vi "GPS.vi"() -> ()   [LabVIEW 2020]
uses:
  <vilib>/Instr/_visa.llb/VISA Configure Serial Port (Instr).vi
panel:
  out "before substring 10":string
  out "before substring 9":string
  out "before substring 8":string
  out "before substring 7":string
  out "before substring 6":string
  out "before substring 5":string
  out "before substring 4":string
  out "before substring 3":string
  out "before substring 2":string
  out "before substring":string
  in  "VISA resource name":refnum<visa-resource-name>
  in  "label":string
  in  "marker color":string
  in  "WebBrowser":refnum<k7>(container)
  in  "Map Format":string(combo)="roadmap"
  in  "Size X":dbl=450.0
  in  "Size Y":dbl=650.0
  in  "Zoom":sgl=16.0 format="%#.1g"
  in  "Longitude":dbl=-1.3070000000000026 format="%#.6g"
  in  "Latitude":dbl=51.4062 format="%#.6g"
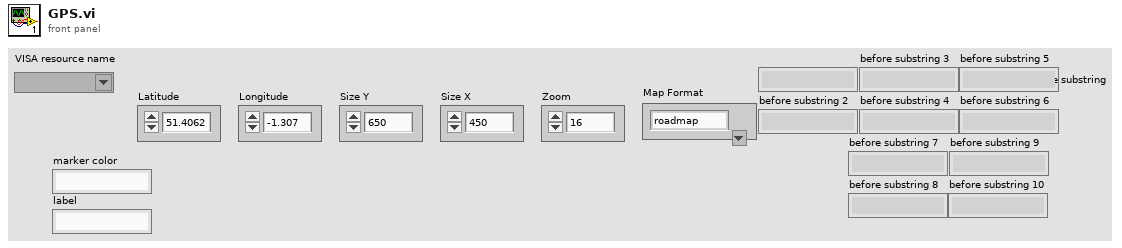
[diagram p1: front panel]
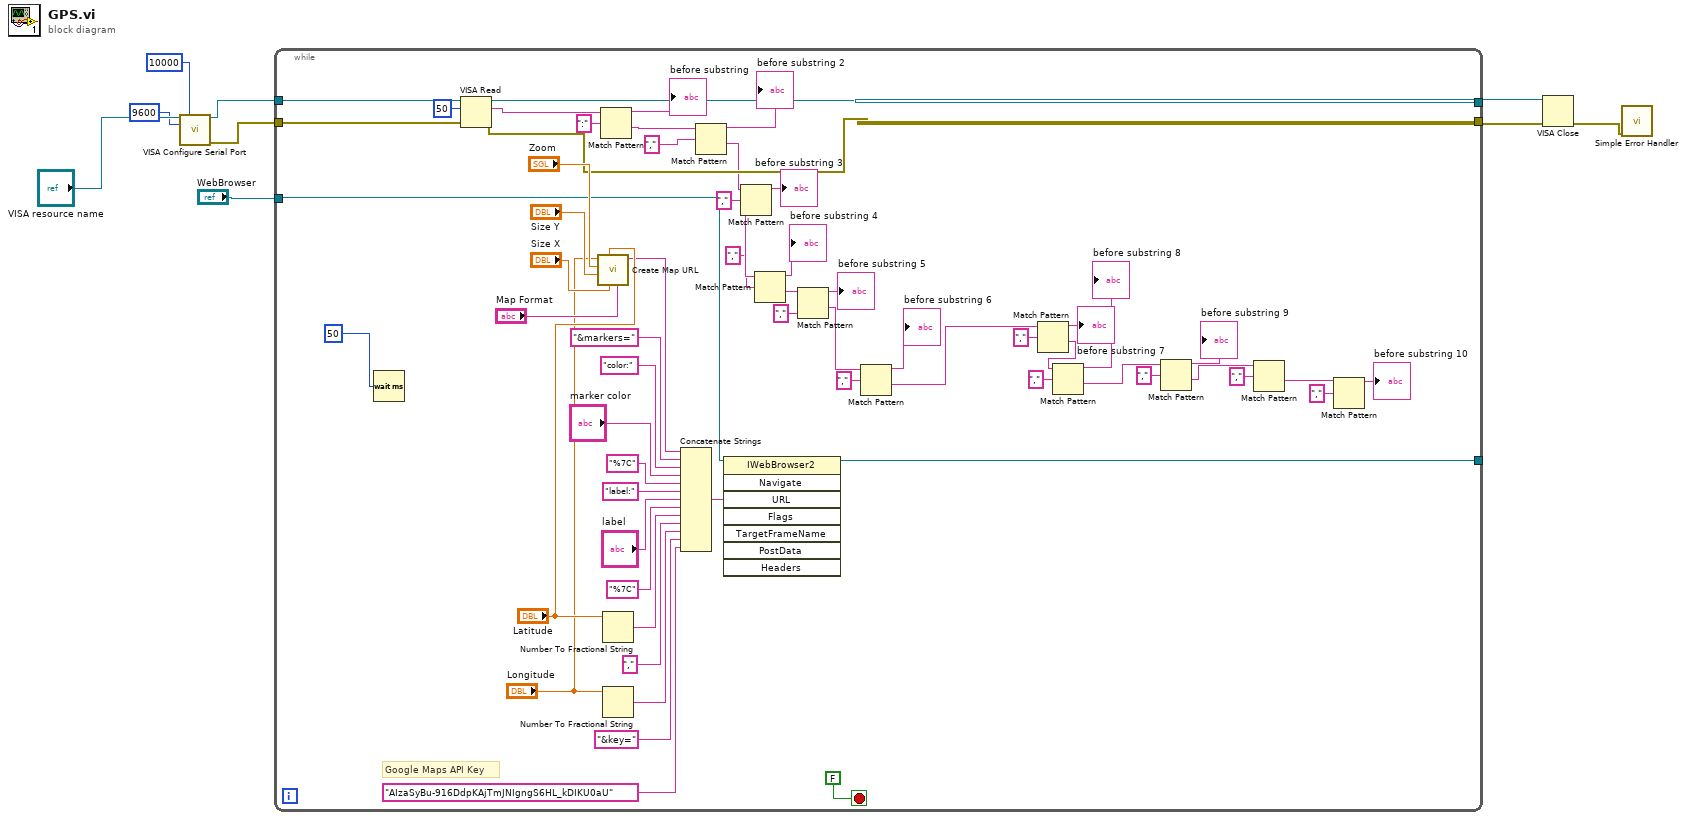
[diagram p0: block diagram]
diagram:
  n1 = call-poly "VISA Configure Serial Port"("VISA resource name"="VISA resource name", "timeout (10sec)"=u32 10000, "baud rate (9600)"=u32 9600) -> ("VISA resource name out"=w1:refnum<visa-resource-name>, "error out"=w6:errorcluster)  [unwired: 11 in]
  n2 = while {
    tunnel: "WebBrowser" -> [w49]
    tunnel: [w48] -> _
    tunnel: [w44] -> w7
    tunnel: w6 -> [w47]
    tunnel: [w46] -> w5
    tunnel: w1 -> [w11]
    stop <- FALSE stop-if-true
    # "Google Maps API Key"
    n3 = Wait (ms)(milliseconds to wait=u32 50) -> ()  [unwired: 1 out]
    n4 = VISA Read(VISA resource name=w11, byte count=u32 50, error in (no error)=w47) -> (VISA resource name out=w44:refnum<visa-resource-name>, read buffer=w45:string, error out=w46:errorcluster)  [unwired: 1 out]
    n5 = call "Create Map URL.vi"("Map Format"="Map Format", "X"="Size X", "Lat"="Latitude", "Y"="Size Y", "Zoom"="Zoom", "Lon"="Longitude") -> ("String"=w42:string)  [unwired: 5 in]
    n6 = Match Pattern(string=w45, regular expression=":") -> (before substring=→"before substring":string, after substring=w41:string)  [unwired: 1 in, 2 out]
    n7 = Number To Fractional String(number="Latitude") -> (F-format string=w56:string)  [unwired: 3 in]
    n8 = Number To Fractional String(number="Longitude") -> (F-format string=w54:string)  [unwired: 3 in]
    n9 = Concatenate Strings(w42, "&markers=" ("string"), "color:" ("string"), "marker color", "%7C" ("string"), "label:" ("string"), "label", "%7C" ("string"), w56, "," ("string"), w54, "&key=" ("string"), "AIzaSyBu-916DdpKAjTmJNIgngS6HL_kDIKU0aU" ("string")) -> (w50:string)
    n10 = Match Pattern(string=w41, regular expression=",") -> (before substring=→"before substring 2":string, after substring=w38:string)  [unwired: 1 in, 2 out]
    n11 = invoke class="IWebBrowser2" method="Navigate"(reference=w49, "URL"=w50) -> (reference out=w48:refnum<k7>)  [unwired: 6 in, 7 out]
    n12 = Match Pattern(string=w38, regular expression=",") -> (before substring=→"before substring 3":string, after substring=w36:string)  [unwired: 1 in, 2 out]
    n13 = Match Pattern(string=w36, regular expression=",") -> (before substring=→"before substring 4":string, after substring=w31:string)  [unwired: 1 in, 2 out]
    n14 = Match Pattern(string=w31, regular expression=",") -> (before substring=→"before substring 5":string, after substring=w28:string)  [unwired: 1 in, 2 out]
    n15 = Match Pattern(string=w28, regular expression=",") -> (before substring=→"before substring 6":string, after substring=w26:string)  [unwired: 1 in, 2 out]
    n16 = Match Pattern(string=w26, regular expression=",") -> (before substring=→"before substring 7":string, after substring=w22:string)  [unwired: 1 in, 2 out]
    n17 = Match Pattern(string=w22, regular expression=",") -> (before substring=→"before substring 8":string, after substring=w19:string)  [unwired: 1 in, 2 out]
    n18 = Match Pattern(string=w19, regular expression=",") -> (before substring=→"before substring 9":string, after substring=w17:string)  [unwired: 1 in, 2 out]
    n19 = Match Pattern(string=w17, regular expression=",") -> (after substring=w14:string)  [unwired: 1 in, 3 out]
    n20 = Match Pattern(string=w14, regular expression=",") -> (before substring=→"before substring 10":string)  [unwired: 1 in, 3 out]
  }
  n21 = VISA Close(VISA resource name=w7, error in (no error)=w5) -> (error out=w2:errorcluster)
  n22 = call <vilib>:"Simple Error Handler.vi"("error in (no error)"=w2) -> ()  [unwired: 4 in, 5 out]
